vi "pre_build.vi"(6 "Top Level/Always Included VIs":path[](array[path]), 7 "Main Destination Path":path, 9 "Target Name":string, 10 "Build Specification Name":string, 11 "Project Path":path) -> (0 "error out":errorcluster)   [LabVIEW 2019]
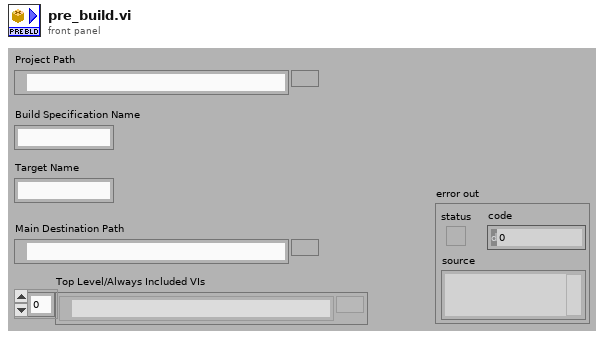
[diagram p1: front panel]
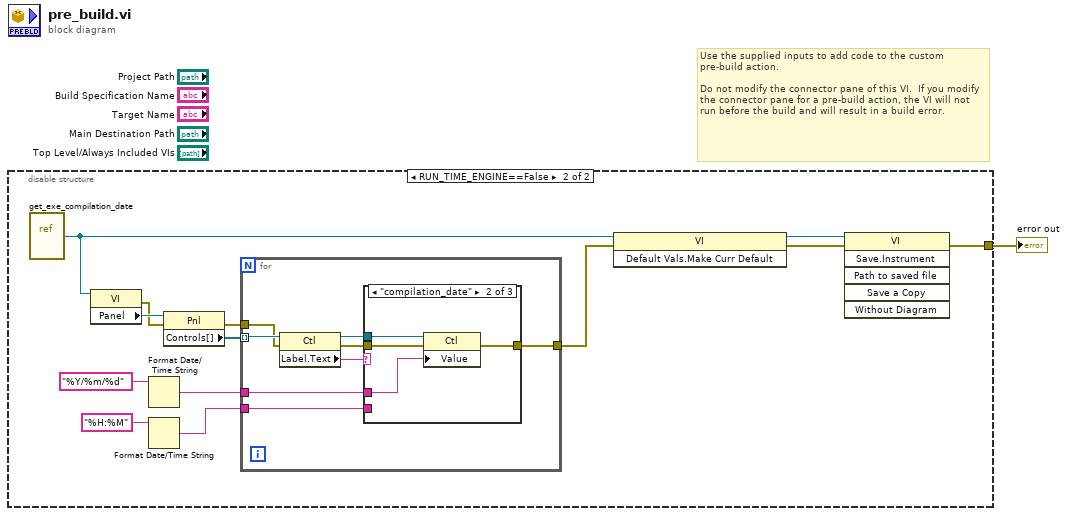
[diagram p0: block diagram]
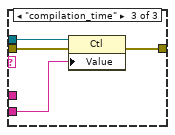
[diagram p4: hidden frame]
diagram:
  # "Use the supplied inputs to add code to the custom pre-build action.\n\nDo not modify the connector pane of this VI.  If you modify the connector pane for a pre-build action, the VI will not run before the build and will result in a build error."
  n1 = disable-structure shown="RUN_TIME_ENGINE==False" {
    disable-tunnel: [_ w6] -> w1
    frame condition #0 {
    }
    frame condition #1 (active) {
      n2 = vi-ref "get_exe_compilation_date.vi"() -> (w12:refnum<vi>)
      n3 = property class="VI"(reference=w12) -> (error out=w11:errorcluster, "Panel"=w14:refnum<vi>)  [unwired: 1 in, 1 out]
      n4 = Format Date/Time String(time format string (%c)="%Y/%m/%d") -> (date/time string=w4:string)  [unwired: 2 in]
      n5 = Format Date/Time String(time format string (%c)="%H:%M") -> (date/time string=w2:string)  [unwired: 2 in]
      n6 = property class="Pnl"(reference=w14, error in=w11) -> (error out=w10:errorcluster, "Controls[]"=w13:refnum<vi>[])  [unwired: 1 out]
      n7 = for {
        tunnel: w13 -> [w22] mode=indexing
        tunnel: w4 -> [w19]
        tunnel: w2 -> [w18]
        tunnel: w10 -> [w17]
        tunnel: [w15] -> w9
        n8 = property class="Ctl"(reference=w22, error in=w17) -> (reference out=w20:refnum<vi>, error out=w16:errorcluster, "Label.Text"=w21:string)
        n9 = case shown="\"compilation_date\"" w21 {
          tunnel: w20 -> [_ w27 w31]
          tunnel: w19 -> [_ w26 _]
          tunnel: w18 -> [_ _ w30]
          tunnel: w16 -> [w23 w25 w29]
          tunnel: [w23 w24 w28] -> w15
          frame Default {
          }
          frame "compilation_date" {
            n10 = property class="Ctl"(reference=w27, error in=w25, "Value"=w26) -> (error out=w24:errorcluster)  [unwired: 1 out]
          }
          frame "compilation_time" {
            n11 = property class="Ctl"(reference=w31, error in=w29, "Value"=w30) -> (error out=w28:errorcluster)  [unwired: 1 out]
          }
        }
      }
      n12 = invoke class="VI" method="Default Vals.Make Curr Default"(reference=w12, error in=w9) -> (reference out=w8:refnum<vi>, error out=w7:errorcluster)  [unwired: 1 in, 1 out]
      n13 = invoke class="VI" method="Save.Instrument"(reference=w8, error in=w7) -> (error out=w6:errorcluster)  [unwired: 4 in, 5 out]
    }
  }
  "error out" <- w1
